vi "Catalogue (Read).vi"(6 "ISOBUS address":T3=-1 caption="ISOBUS address (-1)", 8 "error in":errorcluster, 11 "Mercury Reference In":T4) -> (0 "error out":errorcluster, 2 "Devices":string[](array[string]), 3 "Mercury Reference Out":T4, 4 "Valid?":T2)   [LabVIEW 2019, in "Mercury iXX.lvlib" / "System.lvlib"]
doc: "Read and display the unique identifier of each device in the Mercury System."
uses:
  System.lvlib
  Controls/Mercury Reference.ctl
  CryoTUM_20210311/sub_vi-s/Equipment/Mercury iXX/Public/Controls/Comms Transport Layer.ctl
  Private/Controls/Query Dynamic Reference.ctl
  Controls/ISOBus Address.ctl
  Controls/Is Valid LED.ctl
  Controls/Catalogue.ctl
  Private/Controls/Command Verbs.ctl
  mercury/Mercury iXX.lvlib
panel:
  out "Catalogue":T1
  # "Mainboard"
  # "Daughter Boards"
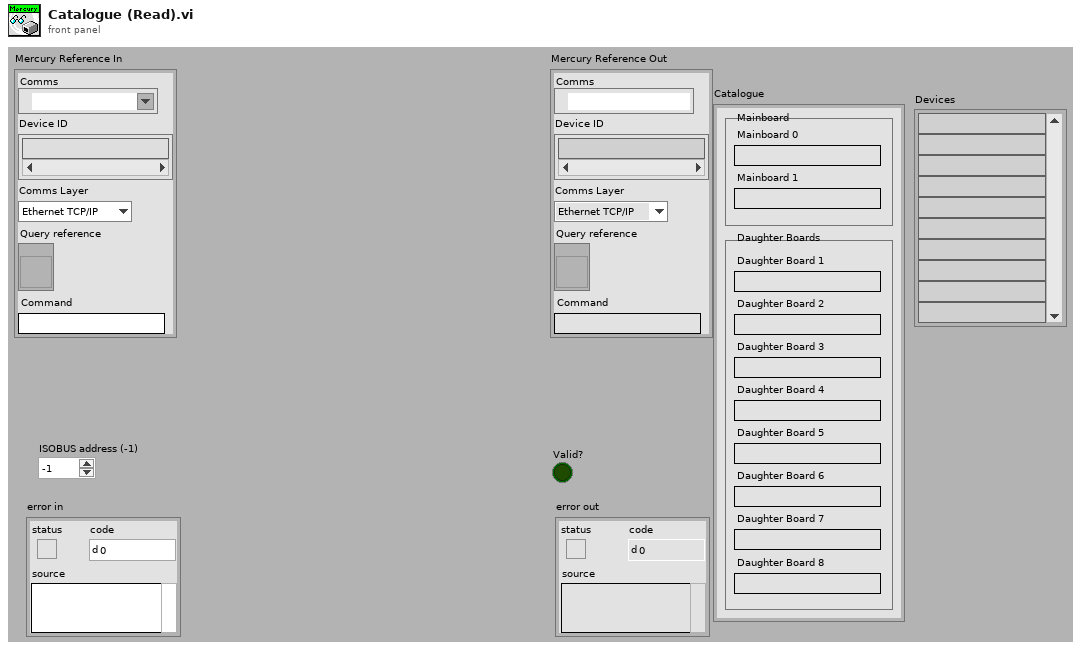
[diagram p1: front panel]
types:
  T1 = typedef "Mercury iXX.lvlib/System.lvlib/Catalogue.ctl" = cluster{"Mainboard 0":string, "Mainboard 1":string, "Daughter Board 1":string, "Daughter Board 2":string, "Daughter Board 3":string, "Daughter Board 4":string, "Daughter Board 5":string, "Daughter Board 6":string, "Daughter Board 7":string, "Daughter Board 8":string}
  T2 = typedef "Mercury iXX.lvlib/Is Valid LED.ctl" = bool
  T3 = typedef "Mercury iXX.lvlib/ISOBus Address.ctl" = i32
  T4 = typedef "Mercury iXX.lvlib/Mercury Reference.ctl" = cluster{"Comms":refnum<visa-resource-name>, "Device ID":string[], "Comms Layer":T5, "Command":string, "Query reference":T6}
  T5 = typedef "Mercury iXX.lvlib/Comms Transport Layer.ctl" = enum16{"Ethernet TCP/IP", "USB", "ISOBus - RS-232", "GPIB"}
  T6 = typedef "Mercury iXX.lvlib/Query Dynamic Reference.ctl" = refnum<vi>
  T7 = typedef "Mercury iXX.lvlib/Command Verbs.ctl" = string
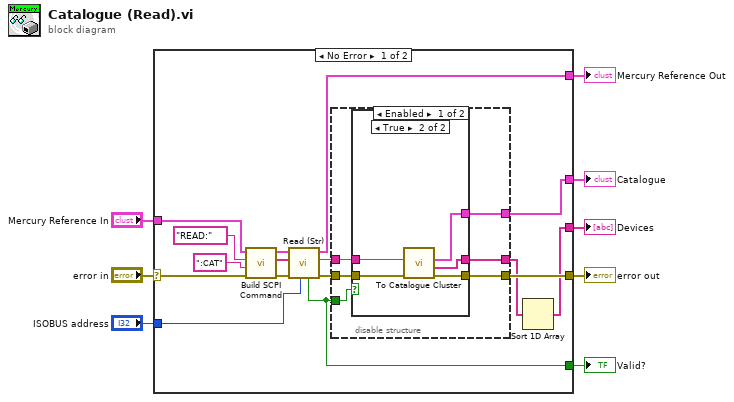
[diagram p0: block diagram]
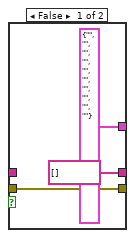
[diagram p2: hidden frame]
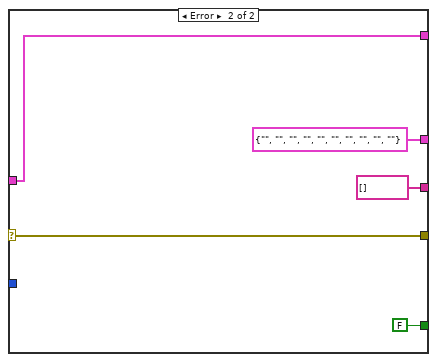
[diagram p4: hidden frame]
diagram:
  n1 = case shown="No Error" "error in" {
    selector: "error in" -> [w11 w42]
    tunnel: "Mercury Reference In" -> [w14 w43]
    tunnel: [w22 w43] -> w7
    tunnel: [w24 w42] -> w6
    tunnel: "ISOBUS address" -> [w18 _]
    tunnel: [w23 T1 {"Mainboard 0"="", "Mainboard 1"="", "Daughter Board 1"="", "Daughter Board 2"="", "Daughter Board 3"="", "Daughter Board 4"="", "Daughter Board 5"="", "Daughter Board 6"="", "Daughter Board 7"="", "Daughter Board 8"=""} ("Catalouge")] -> w2
    tunnel: [w21 FALSE ("Valid?")] -> w3
    tunnel: [w9 string[] [] ("Devices")] -> w1
    frame No Error {
      n2 = call "Build SCPI Command.vi"("error in"=w11, "Noun(s)"=":CAT" ("Command"), "Verb"=T7 "READ:", "Mercury Reference In"=w14) -> ("error out"=w12:errorcluster, "SCPI Message(s)"=w15:string[], "Mercury Reference Out"=w13:T4)  [unwired: 5 out]
      n3 = call "Read (Str).vi"("ISOBUS address"=w18, "error in"=w12, "SCPI Message(s)"=w15, "Mercury Reference In"=w13) -> ("error out"=w19:errorcluster, "Response"=w20:string, "Mercury Reference Out"=w22:T4, "Valid?"=w21:T2)  [unwired: 4 out]
      n4 = disable-structure shown="Enabled" {
        disable-tunnel: w19 -> [w30 _]
        disable-tunnel: [w29 _] -> w24
        disable-tunnel: [w28 _] -> w23
        disable-tunnel: w20 -> [w27 _]
        disable-tunnel: [w26 _] -> w10
        disable-tunnel: w21 -> [w25 _]
        frame Enabled {
          n5 = case shown="True" w25 {
            tunnel: w30 -> [w33 w38]
            tunnel: [w33 w37] -> w29
            tunnel: [T1 {"Mainboard 0"="", "Mainboard 1"="", "Daughter Board 1"="", "Daughter Board 2"="", "Daughter Board 3"="", "Daughter Board 4"="", "Daughter Board 5"="", "Daughter Board 6"="", "Daughter Board 7"="", "Daughter Board 8"=""} ("Catalogue") w36] -> w28
            tunnel: w27 -> [_ w35]
            tunnel: [string[] [] ("Devices") w34] -> w26
            frame False {
            }
            frame True {
              n6 = call "To Catalogue Cluster.vi"("error in"=w38, "Raw Catalogue"=w35) -> ("error out"=w37:errorcluster, "Devices"=w34:string[], "Catalouge"=w36:T1)  [unwired: 7 out]
            }
          }
        }
        frame Disabled {
        }
      }
      n7 = Sort 1D Array(array=w10) -> (sorted array=w9:string[])
    }
    frame Error {
    }
  }
  "Mercury Reference Out" <- w7
  "error out" <- w6
  "Valid?" <- w3
  "Catalogue" <- w2
  "Devices" <- w1
